vi "QGA 6000-1.vi"() -> ()   [LabVIEW 2013]
doc: "This example performs writes and reads on a serial port, as directed by the user. You can press the Write and Read buttons, and change the Read Count, while the example is running.\n\nThe parameters set for the serial port must match the parameters of the connected instrument or device. In this example, the Read Count parameter specifies the number of bytes that the serial port reads. If there were more bytes at the port than the specified number, those bytes would not be read. If there were less bytes at the port than the specified number, you would receive a timeout error.\n\nThis example expands upon the flow control options for XON and XOFF, allowing the user to choose those control characters. Also, the user can enable or disable a termination character. Some devices require a termination character in order to identify the end of command strings. Some devices send a termination character to signify the end of data to be read. This example shows how you can end the Read operation once a termination character is detected in the buffer and/or append a termination character at the end of the Write data."
uses:
  <vilib>/Instr/_visa.llb/VISA Configure Serial Port (Instr).vi
  <vilib>/platform/TimedLoop/XDataNode/XDataNode.xnode
  <vilib>/Platform/TimedLoop/XDataNode/nitl_modes.ctl
  <vilib>/Platform/TimedLoop/XDataNode/XDNodeRunTimeDep.lvlib
  <vilib>/Platform/TimedLoop/XDataNode/wakeup.ctl
  <vilib>/Platform/TimedLoop/XDataNode/timing_clust.ctl
  <vilib>/Utility/file.llb/Write To Spreadsheet File (string).vi
  Program Files/National Instruments/LabVIEW 2013/examples/Instrument IO/Serial/support/Serial - Settings.ctl
panel:
  out "LAMBDA":dbl(graph)
  out "AFR":dbl(graph)
  out "O2 [% ]":dbl(graph)
  out "CO2 [% ]":dbl(graph)
  out "HC [ppm ]":i32(graph)
  out "CO [% ]":dbl(graph)
  in  "NOTA":string
  in  "file path (dialog if empty)":path
  in  "DATO":bool
  out "AFR":dbl format="%.2f"
  out "LAMBDA":dbl format="%.2f"
  out "O2 [ % ]":dbl format="%.2f"
  out "CO2 [ % ]":dbl format="%.2f"
  out "HC [ ppm ]":dbl
  out "CO [ % ]":dbl format="%.2f"
  in  "Stop":bool
  in  "Serial Settings":T1={"baud rate"=9600, "data bits"=8, "parity"=enum."None", "stop bits"=10, "flow control"=0} {"flow control" items=["None"=0, "XON/XOFF"=1, "RTS/CTS"=2, "DTR/DSR"=4]; "stop bits" items=["1.0"=10, "1.5"=15, "2.0"=20]; "data bits" min=5 max=8 step=1; "baud rate" items=["75"=75, "110"=110, "134"=134, "150"=150, "300"=300, "600"=600, "1200"=1200, "1800"=1800, "2400"=2400, "4800"=4800, "7200"=7200, "9600"=9600, "14400"=14400, "19200"=19200, "28800"=28800, "38400"=38400, "56000"=56000, "57600"=57600, "115200"=115200, "128000"=128000, "230400"=230400]}
  in  "VISA resource name":refnum<visa-resource-name>="COM1"
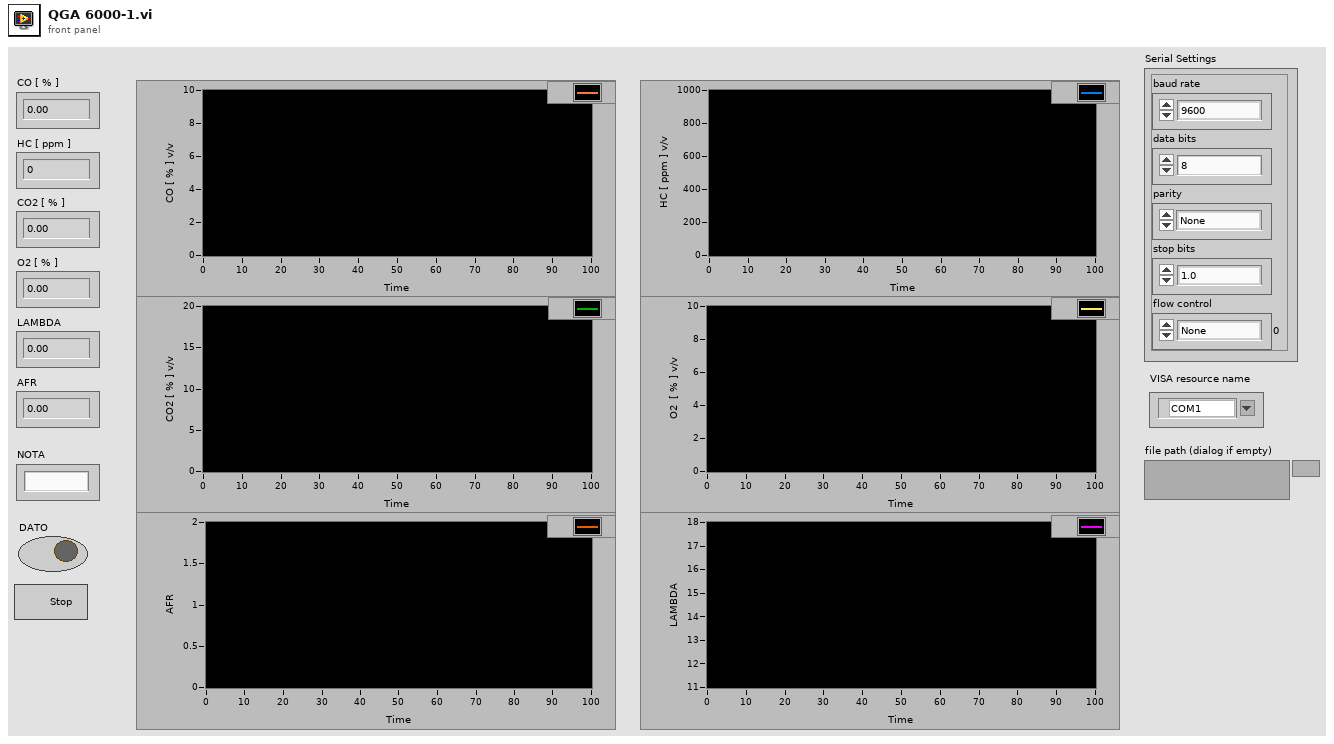
[diagram p1: front panel]
types:
  T1 = typedef "Serial - Settings.ctl" = cluster{"baud rate":u32, "data bits":u16, "parity":enum16{"None", "Odd", "Even", "Mark", "Space"}, "stop bits":u16, "flow control":u16}
  T2 = enum16{"open", "replace", "create", "open or create", "replace or create", "replace or create with confirmation"}
  T3 = typedef "XDNodeRunTimeDep.lvlib/timing_clust.ctl" = cluster{"Expected End [f-1]":u64, "Actual End [f-1]":u64, "Finished Late? [f-1]":bool, "Expected End [i-1]":u64, "Actual End [i-1]":u64, "Finished Late? [i-1]":bool, "Expected Start [i]":u64, "Actual Start [i]":u64, "Expected Start [f]":u64, "Actual Start [f]":u64, "Source Name":string, "Structure Name":string, "Period":i64, "Deadline":i64, "Offset":i64, "Start":i64, "Priority":i32, "Timeout":i32, "Mode":T4, "Wakeup Reason":T5, "Error":errorcluster, "Source Type":string, "Secondary Source Type":string, "Global End Time":u64, "Global Start Time":u64, "Frame Duration":u64, "Iteration Duration":u64, "Assigned CPU":i32, "I/O Scan Engine Mode":u32}
  T4 = typedef "XDNodeRunTimeDep.lvlib/nitl_modes.ctl" = enum32{"No Change", "Process missed periods, maintain original phase", "Discard missed periods, maintain original phase", "Process missed periods, ignore original phase", "Discard missed periods, ignore original phase"}
  T5 = typedef "XDNodeRunTimeDep.lvlib/wakeup.ctl" = enum32{"Normal", "Aborted", "Asynchronous wakeup", "Timing source error", "Timed loop error", "Timeout"}
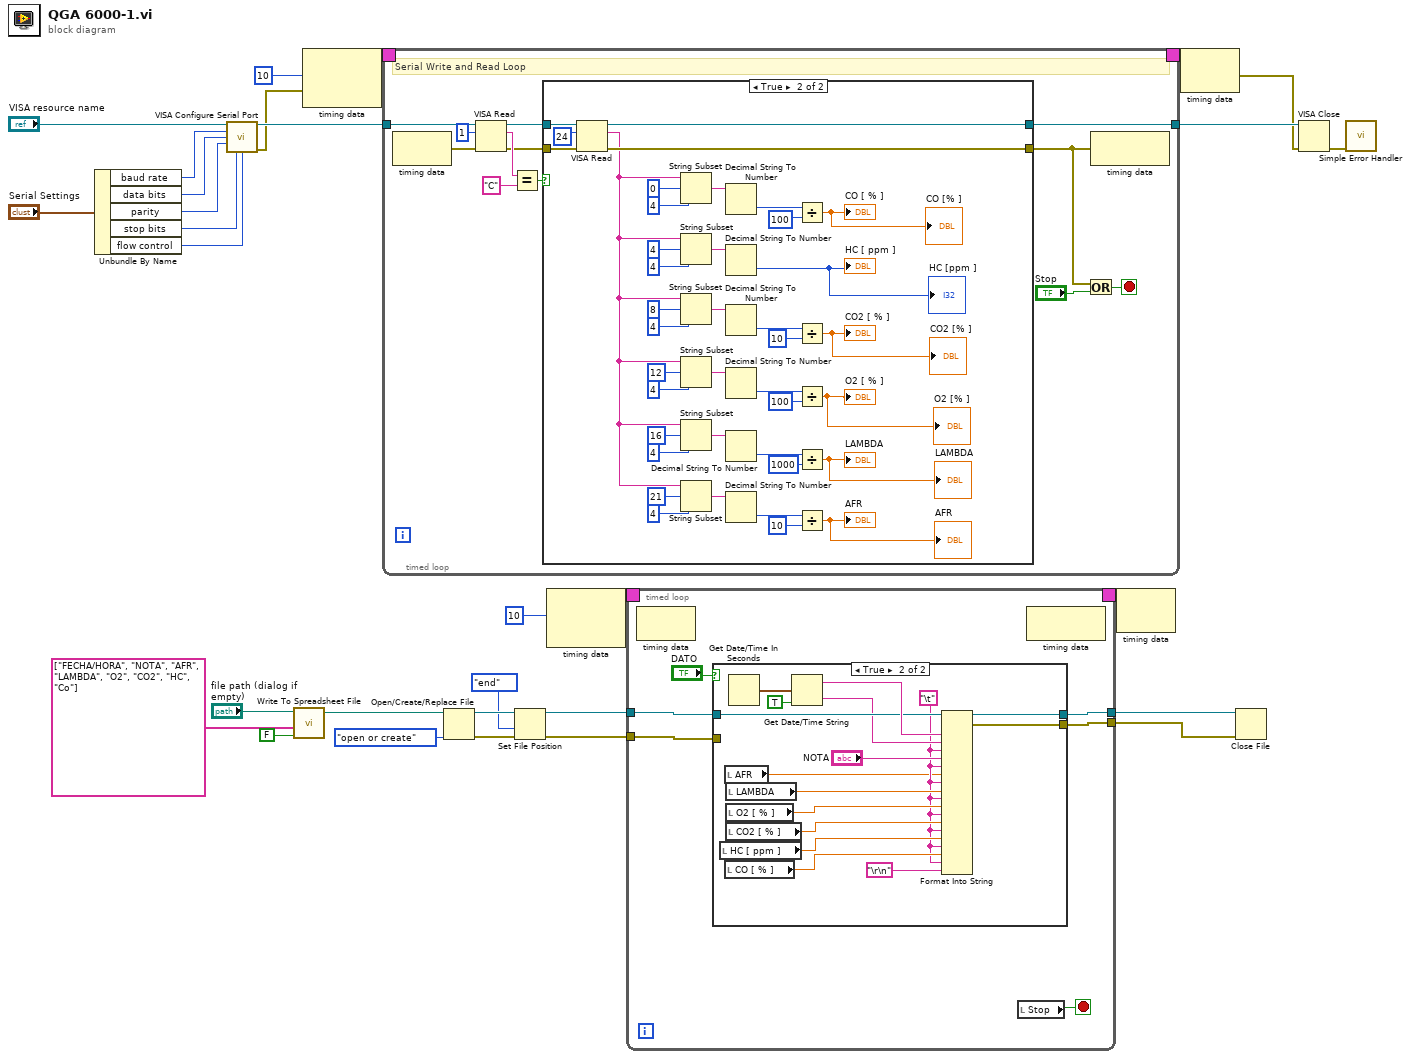
[diagram p0: block diagram]
diagram:
  n1 = Unbundle By Name("Serial Settings") -> ("baud rate"=w26:u32, "data bits"=w27:u16, "parity"=w28:enum16{"None", "Odd", "Even", "Mark", "Space"}, "stop bits"=w29:u16, "flow control"=w23:u16)
  n2 = call-poly "VISA Configure Serial Port"("VISA resource name"="VISA resource name", "baud rate (9600)"=w26, "data bits (8)"=w27, "parity (0:none)"=w28, "stop bits (10: 1 bit)"=w29, "flow control (0:none)"=w23) -> ("VISA resource name out"=w18:refnum<visa-resource-name>, "error out"=w17:errorcluster)  [unwired: 4 in, 4 out]
  n3 = call-poly <vilib>:"Write To Spreadsheet File.vi"("append to file? (new file:F)"=FALSE, "1D data"=string[] ["FECHA/HORA", "NOTA", "AFR", "LAMBDA", "O2", "CO2", "HC", "Co"], "file path (dialog if empty)"="file path (dialog if empty)") -> ("new file path (Not A Path if cancelled)"=w5:path)  [unwired: 5 in]
  n4 = node-c288(i64 10 ("Period"), w17) -> (w21:T3)
  n5 = timed-loop {
    tunnel: [w42] -> w24
    timing: w21 -> [_]
    timing-out: [_] -> w20
    tunnel: w18 -> [w36]
    stop <- w41 stop-if-true
    # "Serial Write and Read Loop"
    n6 = node-c288() -> (w35:errorcluster)  [unwired: 1 in]
    n7 = VISA Read(VISA resource name=w36, byte count=u32 1, error in (no error)=w35) -> (VISA resource name out=w34:refnum<visa-resource-name>, read buffer=w38:string, error out=w33:errorcluster)  [unwired: 1 out]
    n8 = Equal?(x=w38, y="C") -> (x = y?=w32:bool)
    n9 = case shown="True" w32 {
      tunnel: [w44 w84] -> w42
      tunnel: [w43 w83] -> w31
      tunnel: w34 -> [w44 w82]
      tunnel: w33 -> [w43 w81]
      frame False {
      }
      frame True {
        n10 = VISA Read(VISA resource name=w82, byte count=u32 24, error in (no error)=w81) -> (VISA resource name out=w84:refnum<visa-resource-name>, read buffer=w67:string, error out=w83:errorcluster)  [unwired: 1 out]
        n11 = String Subset(string=w67, offset (0)=0, length (rest)=4 ("length (rest)")) -> (substring=w66:string)
        n12 = String Subset(string=w67, offset (0)=4, length (rest)=4 ("length (rest)")) -> (substring=w65:string)
        n13 = String Subset(string=w67, offset (0)=8, length (rest)=4 ("length (rest)")) -> (substring=w64:string)
        n14 = String Subset(string=w67, offset (0)=12, length (rest)=4 ("length (rest)")) -> (substring=w63:string)
        n15 = String Subset(string=w67, offset (0)=16, length (rest)=4 ("length (rest)")) -> (substring=w62:string)
        n16 = String Subset(string=w67, offset (0)=21, length (rest)=4 ("length (rest)")) -> (substring=w61:string)
        n17 = Decimal String To Number(string=w66) -> (number=w60:i32)  [unwired: 2 in, 1 out]
        n18 = Decimal String To Number(string=w65) -> (number=→"HC [ ppm ]" →"HC [ppm ]":i32)  [unwired: 2 in, 1 out]
        n19 = Decimal String To Number(string=w64) -> (number=w57:i32)  [unwired: 2 in, 1 out]
        n20 = Decimal String To Number(string=w63) -> (number=w55:i32)  [unwired: 2 in, 1 out]
        n21 = Decimal String To Number(string=w62) -> (number=w53:i32)  [unwired: 2 in, 1 out]
        n22 = Decimal String To Number(string=w61) -> (number=w51:i32)  [unwired: 2 in, 1 out]
        n23 = Divide(x=w60, y=100) -> (x/y=→"CO [ % ]" →"CO [% ]":dbl)
        n24 = Divide(x=w57, y=10) -> (x/y=→"CO2 [ % ]" →"CO2 [% ]":dbl)
        n25 = Divide(x=w55, y=100) -> (x/y=→"O2 [ % ]" →"O2 [% ]":dbl)
        n26 = Divide(x=w53, y=1000) -> (x/y=→"LAMBDA" →"LAMBDA":dbl)
        n27 = Divide(x=w51, y=10) -> (x/y=→"AFR" →"AFR":dbl)
      }
    }
    n28 = Or(x=w31, y="Stop") -> (x .or. y?=w41:bool)
    n29 = node-c288(w31) -> ()  [unwired: 1 out]
  }
  n30 = Open/Create/Replace File(file path (use dialog)=w5, operation (0:open)=T2."open or create") -> (refnum out=w9:refnum<file>, error out=w8:errorcluster)  [unwired: 4 in, 1 out]
  n31 = Set File Position(refnum=w9, from (0:start)=enum16{"start", "end", "current"}."end", error in=w8) -> (refnum out=w4:refnum<file>, error out=w3:errorcluster)  [unwired: 1 in]
  n32 = node-c288(i64 10 ("Period")) -> (w12:T3)  [unwired: 1 in]
  n33 = timed-loop {
    timing: w12 -> [_]
    timing-out: [_] -> w11
    tunnel: w4 -> [w93]
    tunnel: w3 -> [w92]
    tunnel: [w91] -> w2
    tunnel: [w90] -> w1
    stop <- w94 stop-if-true
    n34 = node-c288() -> ()  [unwired: 1 in, 1 out]
    n35 = case shown="True" "DATO" {
      tunnel: w93 -> [w99 w113]
      tunnel: w92 -> [w98 _]
      tunnel: [w99 w112] -> w91
      tunnel: [w98 w111] -> w90
      frame False {
      }
      frame True {
        w103 = "\t"
        n36 = local read "HC [ ppm ]"() -> (w105:dbl)
        n37 = local read "AFR"() -> (w100:dbl)
        n38 = local read "CO [ % ]"() -> (w104:dbl)
        n39 = local read "LAMBDA"() -> (w108:dbl)
        n40 = local read "O2 [ % ]"() -> (w107:dbl)
        n41 = local read "CO2 [ % ]"() -> (w106:dbl)
        n42 = Get Date/Time In Seconds() -> (seconds since 1Jan1904=w114:timestamp)
        n43 = Get Date/Time String(seconds (now)=w114, want seconds? (F)=TRUE) -> (date string=w115:string, time string=w110:string)  [unwired: 1 in]
        n44 = Format Into String(initial string=w113, w115, w110, w103, "NOTA", w103, w100, w103, w108, w103, w107, w103, w106, w103, w105, w103, w104, w103, "\r\n") -> (resulting string=w112:refnum<file>, error out=w111:errorcluster)  [unwired: 2 in]
      }
    }
    n45 = local read "Stop"() -> (w94:bool)
    n46 = node-c288() -> ()  [unwired: 1 in, 1 out]
  }
  n47 = node-c288(w11) -> ()  [unwired: 1 out]
  n48 = node-c288(w20) -> (w16:errorcluster)
  n49 = Close File(refnum=w2, error in=w1) -> ()  [unwired: 2 out]
  n50 = VISA Close(VISA resource name=w24, error in (no error)=w16) -> (error out=w22:errorcluster)
  n51 = call <vilib>:"Simple Error Handler.vi"("error in (no error)"=w22) -> ()  [unwired: 1 in, 8 out]
